vi "backup_Syringe Heaters.vi"   [LabVIEW 2015]
uses:
  <vilib>/eio/EIONode/EIONode.xnode
  <vilib>/rvi/eio/common/nirviEmuTemplateMethod_errors.vi
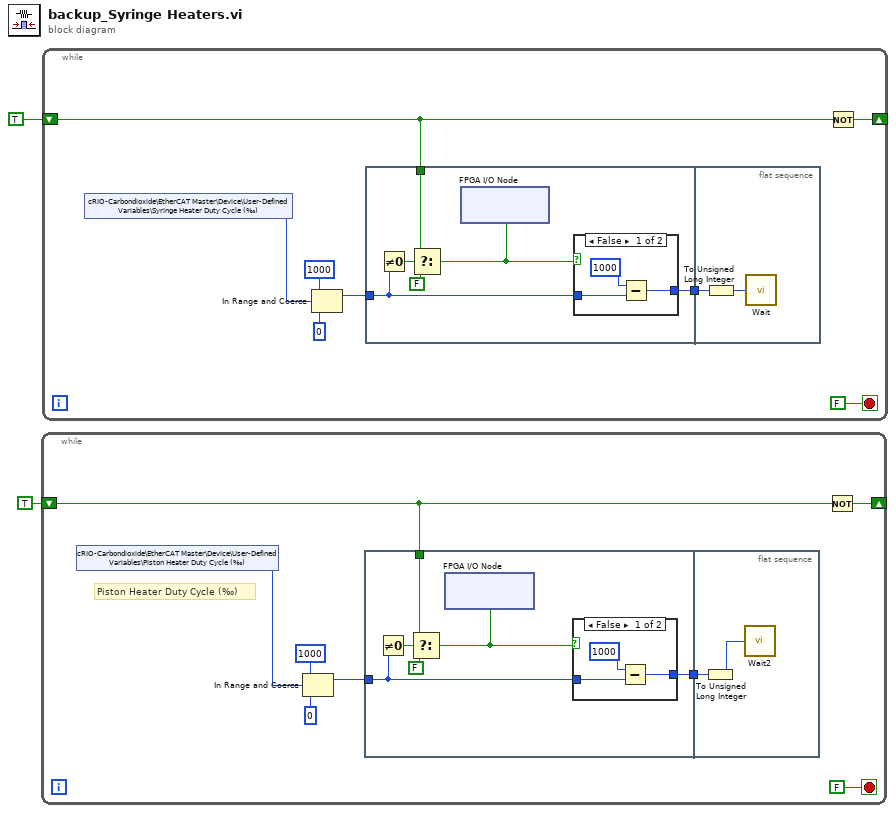
[diagram p0: block diagram]
diagram:
  n1 = while {
    shift-right: [w8] -> _
    shift-left: TRUE -> [w7]
    stop <- FALSE stop-if-true
    # "Piston Heater Duty Cycle (‰)"
    n2 = shared-variable "cRIO-Carbondioxide\\EtherCAT Master\\Device\\User-Defined Variables\\Piston Heater Duty Cycle (‰)"() -> (w3:i16)  [unwired: 1 in, 1 out]
    n3 = In Range and Coerce(upper limit=i16 1000, x=w3, lower limit=i16 0) -> (coerced(x)=w4:i16)  [unwired: 1 out]
    n4 = flat-sequence {
      tunnel: w7 -> [w14]
      tunnel: w4 -> [w12]
      tunnel: [w16] -> w6
      tunnel: w6 -> [w22]
      frame #0 {
        n5 = Not Equal To 0?(x=w12) -> (x != 0?=w15:bool)
        n6 = Select(t=w14, s=w15, f=FALSE) -> (s? t:f=w11:bool)
        n7 = xnode "FPGA I/O Node"("Heater A"=w11) -> ()  [unwired: 1 in, 1 out]
        n8 = case shown="False" w11 {
          tunnel: w12 -> [w18 w20]
          tunnel: [w19 w20] -> w16
          frame False {
            n9 = Subtract(x=i16 1000, y=w18) -> (x-y=w19:i16)
          }
          frame True {
          }
        }
      }
      frame #1 {
        n10 = To Unsigned Long Integer(number=w22) -> (unsigned 32bit integer=w21:u32)
        n11 = call "Wait2"("Count(mSec)"=w21) -> ()  [unwired: 1 out]
      }
    }
    n12 = Not(x=w7) -> (.not. x?=w8:bool)
  }
  n13 = while {
    shift-right: [w28] -> _
    shift-left: TRUE -> [w27]
    stop <- FALSE stop-if-true
    n14 = shared-variable "cRIO-Carbondioxide\\EtherCAT Master\\Device\\User-Defined Variables\\Syringe Heater Duty Cycle (‰)"() -> (w23:i16)  [unwired: 1 in, 1 out]
    n15 = In Range and Coerce(upper limit=i16 1000, x=w23, lower limit=i16 0) -> (coerced(x)=w24:i16)  [unwired: 1 out]
    n16 = flat-sequence {
      tunnel: w27 -> [w34]
      tunnel: w24 -> [w31]
      tunnel: [w36] -> w26
      tunnel: w26 -> [w42]
      frame #0 {
        n17 = Not Equal To 0?(x=w31) -> (x != 0?=w35:bool)
        n18 = Select(t=w34, s=w35, f=FALSE) -> (s? t:f=w32:bool)
        n19 = xnode "FPGA I/O Node"("Heater B"=w32) -> ()  [unwired: 1 in, 1 out]
        n20 = case shown="False" w32 {
          tunnel: w31 -> [w38 w40]
          tunnel: [w39 w40] -> w36
          frame False {
            n21 = Subtract(x=i16 1000, y=w38) -> (x-y=w39:i16)
          }
          frame True {
          }
        }
      }
      frame #1 {
        n22 = To Unsigned Long Integer(number=w42) -> (unsigned 32bit integer=w41:u32)
        n23 = call "Wait"("Count(mSec)"=w41) -> ()  [unwired: 1 out]
      }
    }
    n24 = Not(x=w27) -> (.not. x?=w28:bool)
  }
